vi "NILIA_9233fs.vi"(11 "Data Rate":T1=2 items=["50.000 kS/s (NI 9233)"=2, "33.333 kS/s (NI 9233)"=3, "25.000 kS/s (NI 9233)"=34, "16.667 kS/s (NI 9233)"=35, "12.500 kS/s (NI 9233)"=36, "10.000 kS/s (NI 9233)"=37, "  8.333 kS/s (NI 9233)"=38, "  7.143 kS/s (NI 9233)"=39, "  6.250 kS/s (NI 9233)"=40, "  5.556 kS/s (NI 9233)"=41, "  5.000 kS/s (NI 9233)"=42, "  4.545 kS/s (NI 9233)"=43, "  4.167 kS/s (NI 9233)"=44, "  3.846 kS/s (NI 9233)"=45, "  3.571 kS/s (NI 9233)"=46, "  3.333 kS/s (NI 9233)"=47, "  3.125 kS/s (NI 9233)"=48, "  2.941 kS/s (NI 9233)"=49, "  2.778 kS/s (NI 9233)"=50, "  2.632 kS/s (NI 9233)"=51, "  2.500 kS/s (NI 9233)"=52, "  2.381 kS/s (NI 9233)"=53, "  2.273 kS/s (NI 9233)"=54, "  2.174 kS/s (NI 9233)"=55, "  2.083 kS/s (NI 9233)"=56, "  2.000 kS/s (NI 9233)"=57]) -> (3 "fs":dbl)   [LabVIEW 2016]
uses:
  <vilib>/LabVIEW Targets/FPGA/cRIO/shared/nicrio_ModuleControls/nicrio_cRIO-9233_DataRatesRing.ctl
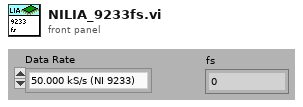
[diagram p1: front panel]
types:
  T1 = typedef "nicrio_cRIO-9233_DataRatesRing.ctl" = u8
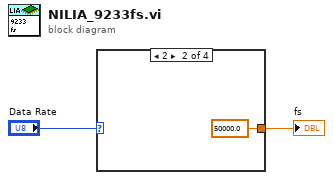
[diagram p0: block diagram]
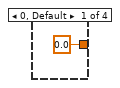
[diagram p2: hidden frame]
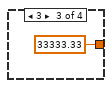
[diagram p3: hidden frame]
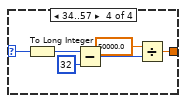
[diagram p4: hidden frame]
diagram:
  n1 = case shown="2" "Data Rate" {
    selector: "Data Rate" -> [_ _ _ w11]
    tunnel: [0.0 50000.0 33333.33 w9] -> w1
    frame 0, Default {
    }
    frame 2 {
    }
    frame 3 {
    }
    frame 34..57 {
      n2 = To Long Integer(number=w11) -> (32bit integer=w8:i32)
      n3 = Subtract(x=w8, y=32) -> (x-y=w6:i32)
      n4 = Divide(x=50000.0, y=w6) -> (x/y=w9:dbl)
    }
  }
  "fs" <- w1
